vi "Read hist cluster element.vi"(7 "Hist cluster element":i32, 8 "error in (no error)":errorcluster, 9 "Secondary":i8=-1, 10 "Primary":i8=-1, 11 "histogram in":T1) -> (0 "error out":errorcluster, 2 "histogram":T2 {"S:" format="%_3f"}, 3 "histogram out":T1)   [LabVIEW 2016]
uses:
  Typedefs/Coincidence single histogram.ctl
  Typedefs/Coincidence histogram cluster refnum.ctl
panel:
  # "You can specify the histogram you want either by giving the index\nin the cluster (hist cluster element), or by specifying the primary and\nsecondary channel that the histogram corresponds to.\n\nIf you leave Primary and Secondary blank, it will use Hist cluster element."
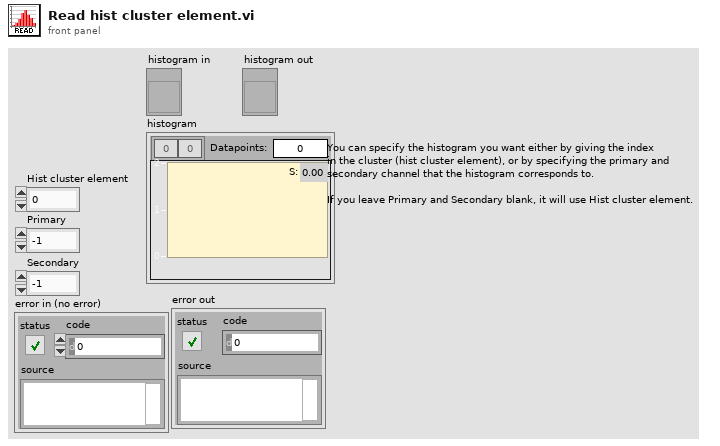
[diagram p1: front panel]
types:
  T1 = typedef "Coincidence histogram cluster refnum.ctl" = refnum<vi>
  T2 = typedef "Coincidence single histogram.ctl" = cluster{"Histogram Graph":cluster{"X Values":dbl[], "Histogram: h(x)":i32[]}[], "IDs":i8[], "Datapoints:":i32, "S:":dbl, "Data array":cluster{"Data":i32[], "Max index":i32, "Current index":i32, "Numofpoints":i32}}
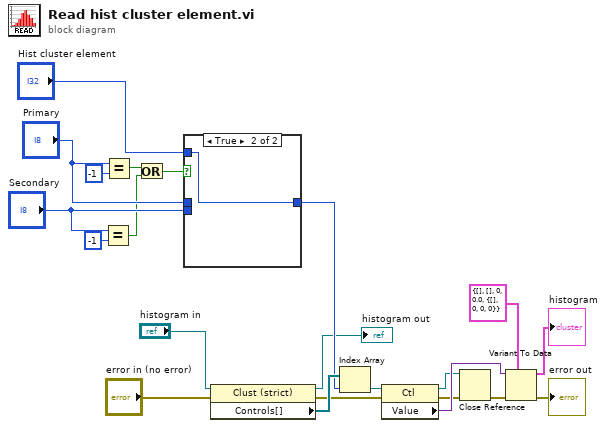
[diagram p0: block diagram]
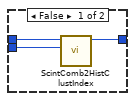
[diagram p2: hidden frame]
diagram:
  n1 = Equal?(x="Secondary", y=-1) -> (x = y?=w5:bool)
  n2 = Equal?(x="Primary", y=-1) -> (x = y?=w6:bool)
  n3 = Or(x=w6, y=w5) -> (x .or. y?=w4:bool)
  n4 = case shown="True" w4 {
    tunnel: "Primary" -> [w25 _]
    tunnel: "Secondary" -> [w24 _]
    tunnel: [w23 w26] -> w21
    tunnel: "Hist cluster element" -> [_ w26]
    frame False {
      n5 = call "ScintComb2HistClustIndex.vi"("Secondary"=w24, "Primary"=w25) -> ("Numeric"=w23:i32)  [unwired: 9 in]
    }
    frame True {
    }
  }
  n6 = property class="Clust (strict)"(reference="histogram in", error in="error in (no error)") -> (reference out=→"histogram out":T1, error out=w16:errorcluster, "Controls[]"=w22:refnum<vi>[])
  n7 = Index Array(array=w22, index=w21) -> (element=w20:refnum<vi>)
  n8 = property class="Ctl"(reference=w20, error in=w16) -> (reference out=w13:refnum<vi>, error out=w14:errorcluster, "Value"=w19:variant)
  n9 = Close Reference(reference=w13, error in (no error)=w14) -> (error out=w12:errorcluster)
  n10 = Variant To Data(error in=w12, type=T2 {"Histogram Graph"=[], "IDs"=[], "Datapoints:"=0, "S:"=0.0, "Data array"={"Data"=[], "Max index"=0, "Current index"=0, "Numofpoints"=0}} ("Cluster"), Variant=w19) -> (data=→"histogram":T2, error out=→"error out":errorcluster)
